vi "边沿计数.vi"() -> ()   [LabVIEW 2013]
doc: "This example demonstrates how to count the pulse's edges."
uses:
  <userlib>/ArtDAQ/_SubVI/ArtDAQ_CreateCICountEdgesChan.vi
  <userlib>/ArtDAQ/_SubVI/ArtDAQ_Read Counter U32 1Samp.vi
panel:
  out "?":u32
  in  "计数器":string="Dev1/CTR0"
  in  "停止":bool
  out "错误输出":errorcluster
  # "通道属性"
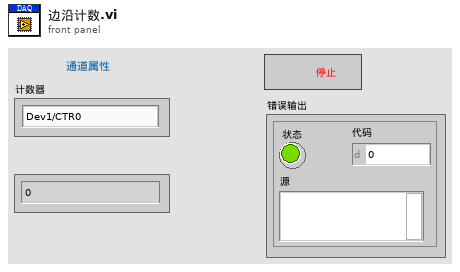
[diagram p1: front panel]
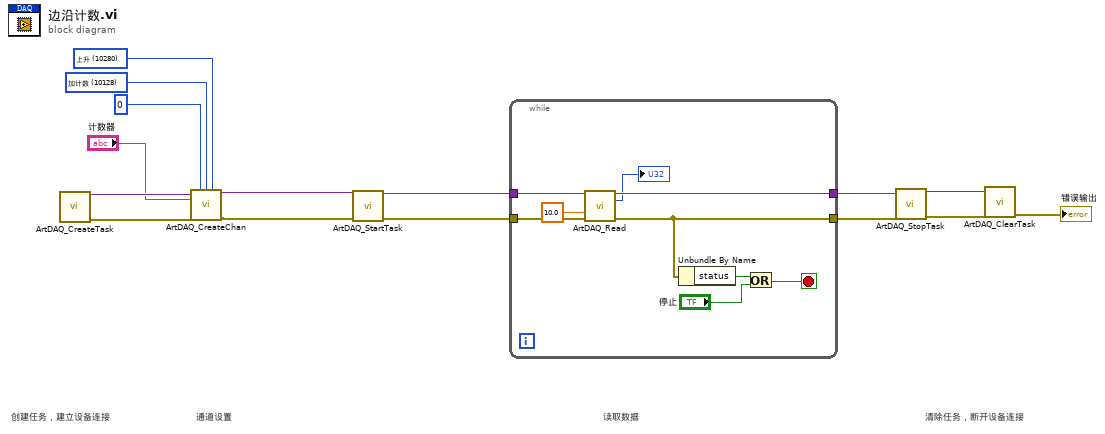
[diagram p0: block diagram]
diagram:
  w11 = 10280 items=["上升"=10280, "下降"=10171] ("Edge")
  w12 = 10128 items=["加计数"=10128, "减计数"=10124, "外部控制"=10326] ("CountDir")
  # "创建任务，建立设备连接"
  # "通道设置"
  # "读取数据"
  # "清除任务，断开设备连接"
  n1 = call <userlib>:"ArtDAQ_CreateTask.vi"() -> ("任务句柄"=w15:variant, "错误输出"=w14:errorcluster)  [unwired: 14 in]
  n2 = call-poly <userlib>:"ArtDAQ_CreateChan.vi"("任务句柄"=w15, "初始计数"=u32 0 ("InitialCount"), "计数方向"=w12, "边沿"=w11, "计数器"="计数器", "错误输入"=w14) -> ("任务句柄"=w2:variant, "错误输出"=w1:errorcluster)  [unwired: 8 in]
  n3 = call <userlib>:"ArtDAQ_StartTask.vi"("任务句柄"=w2, "错误输入"=w1) -> ("任务句柄"=w4:variant, "错误输出"=w3:errorcluster)  [unwired: 12 in]
  n4 = while {
    tunnel: [w24] -> w9
    tunnel: [w20] -> w7
    tunnel: w4 -> [w23]
    tunnel: w3 -> [w22]
    stop <- w17 stop-if-true
    n5 = call-poly <userlib>:"ArtDAQ_Read.vi"("任务句柄"=w23, "超时s"=10.0 ("Timeout"), "错误输入"=w22) -> ("任务句柄"=w24:variant, "数据"=→"?":u32, "错误输出"=w20:errorcluster)  [unwired: 10 in]
    n6 = Unbundle By Name(w20) -> ("status"=w19:bool)
    n7 = Or(x=w19, y="停止") -> (x .or. y?=w17:bool)
  }
  n8 = call <userlib>:"ArtDAQ_StopTask.vi"("任务句柄"=w9, "错误输入"=w7) -> ("任务句柄"=w8:variant, "错误输出"=w6:errorcluster)  [unwired: 12 in]
  n9 = call <userlib>:"ArtDAQ_ClearTask.vi"("任务句柄"=w8, "错误输入"=w6) -> ("错误输出"=→"错误输出":errorcluster)  [unwired: 13 in]
